vi "loadM100CRH3605MDB.vi"() -> ()   [LabVIEW 2012]
uses:
  <vilib>/addons/database/Connection.llb/DB Tools Open Connec (Path).vi
  <vilib>/addons/database/Connection.llb/Conn Execute.vi
  <vilib>/addons/database/Recordset.llb/Rec Destroy - Connection.vi
  <vilib>/addons/database/Connection.llb/DB Tools Open Connec (String).vi
  <vilib>/addons/database/Recordset.llb/Rec Fetch Recordset Data (R).vi
  <vilib>/addons/database/_DB Variant To Data/Database Variant To Data.xnode
  <vilib>/addons/database/NI_Database_API.lvlib
panel:
  out "String":string
  out "concatenated string":string
  out "error out 2":errorcluster
  out "text":string
  in  "path":path=path "C:/temp/mdb"
  out "filenames":string[](array[string])
  out "error out":errorcluster
  in  "Cluster":T1
  out "recordset data":variant[][](array[variant])
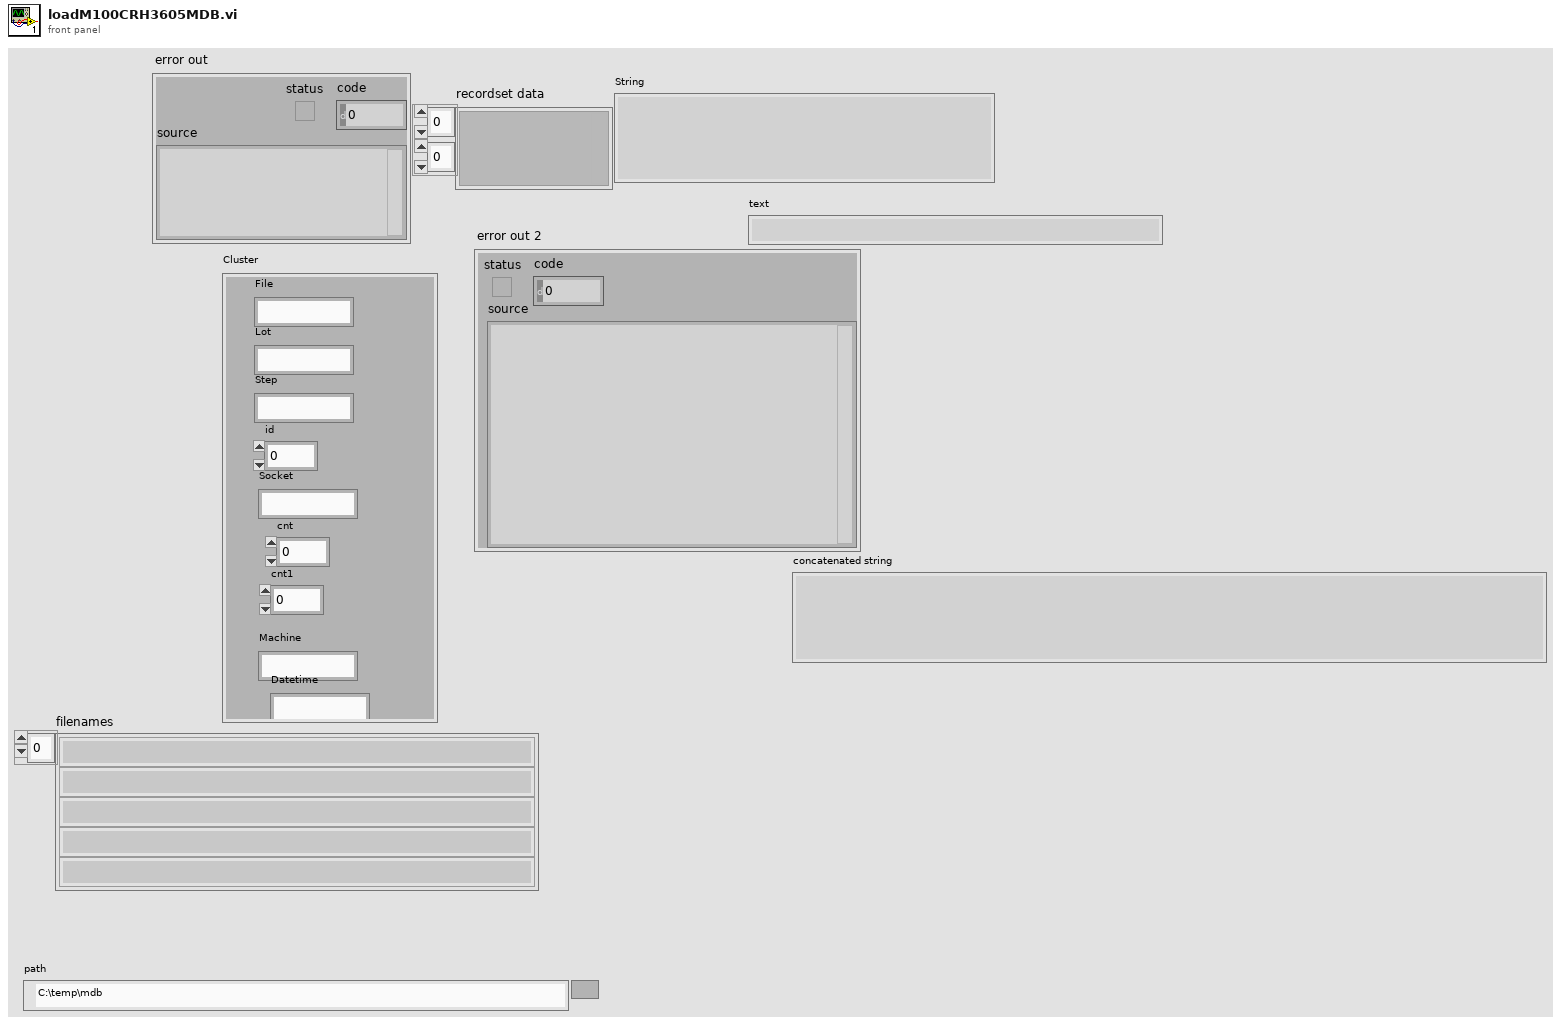
[diagram p1: front panel]
types:
  T1 = cluster{"File":string, "Lot ":string, "Step ":string, "id":dbl, "Socket":string, "cnt":dbl, "cnt1":dbl, "Machine":string, "Datetime":string}
  T2 = typedef "NI_Database_API.lvlib/Conn ObjectReference.ctl" = refnum<k1>
  T3 = typedef "NI_Database_API.lvlib/Rec ObjectReference.ctl" = refnum<k1>
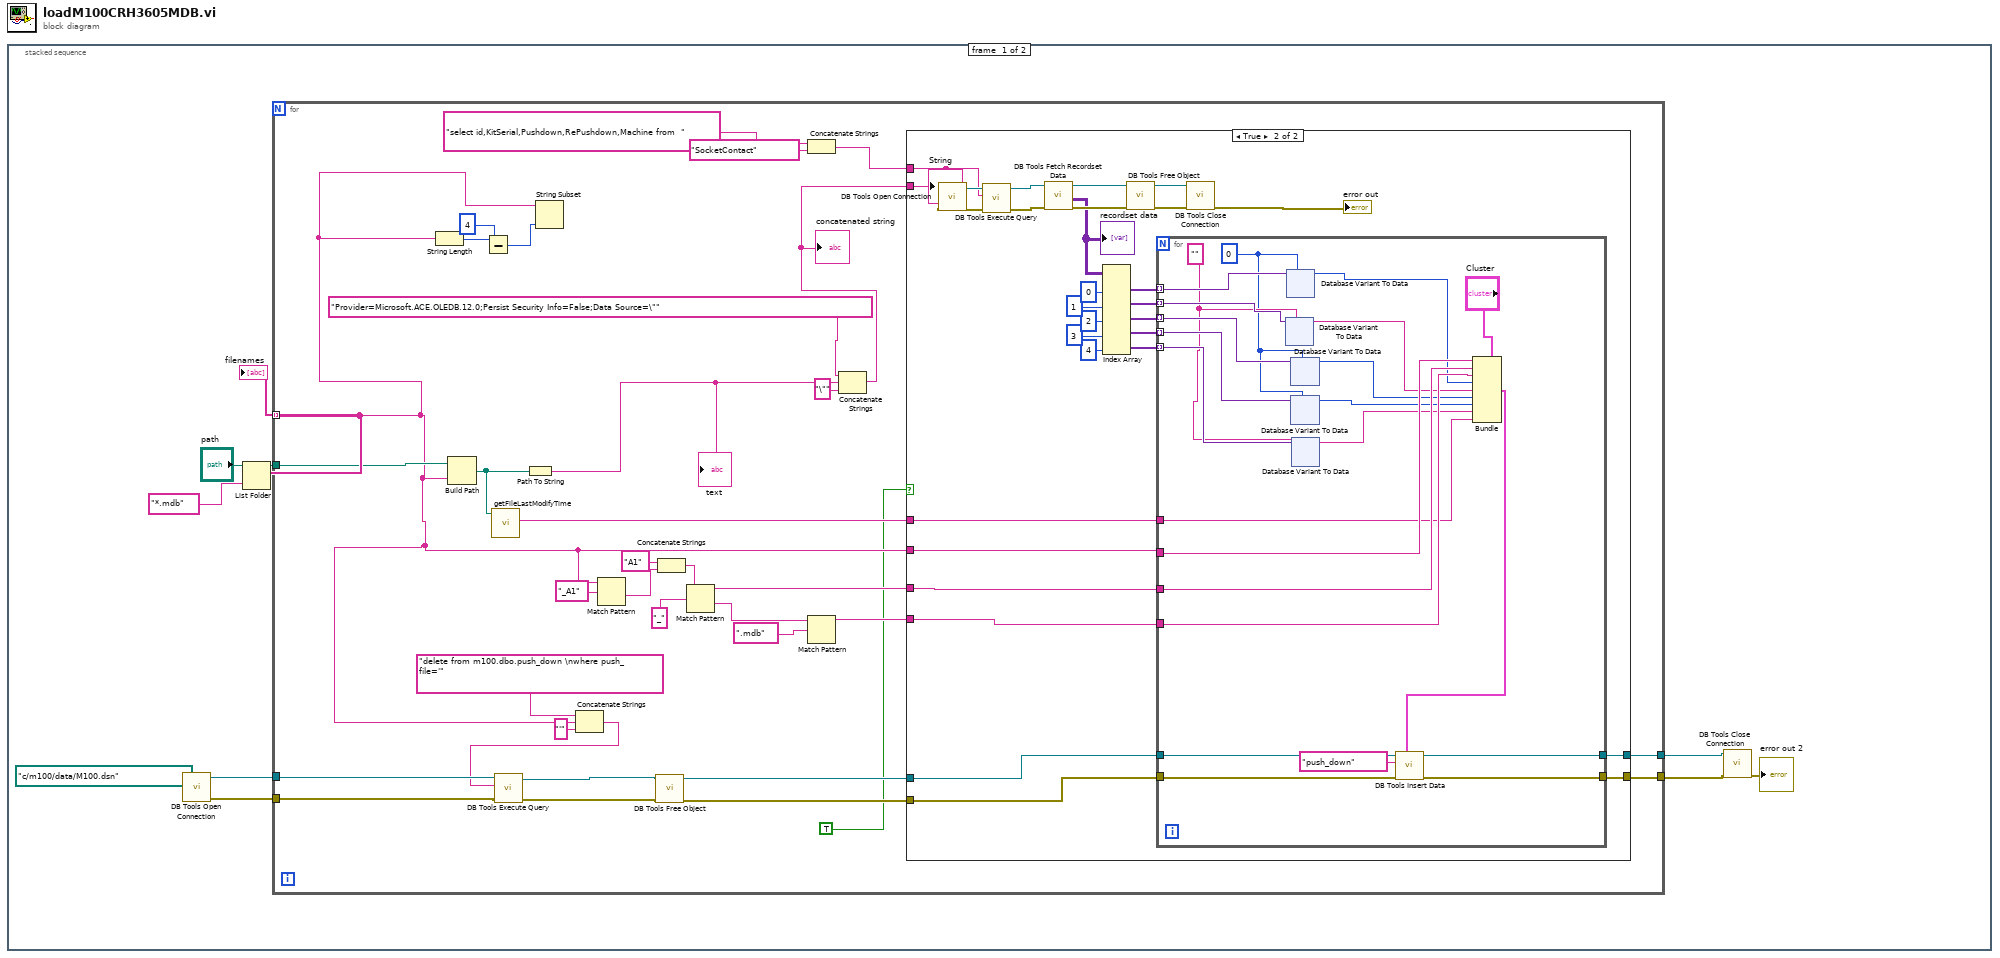
[diagram p0: block diagram]
diagram:
  n1 = stacked-sequence {
    frame #0 {
      n2 = call-poly <vilib>:"DB Tools Open Connection.vi"("connection information"=path "c:/m100/data/M100.dsn") -> ("error out"=w4:errorcluster, "connection reference"=w5:T2)  [unwired: 7 in]
      n3 = List Folder(path="path", pattern="*.mdb") -> (path out=w7:path, filenames=w8:string[])  [unwired: 2 in, 2 out]
      "filenames" <- w8
      n4 = for {
        tunnel: w8 -> [w28] mode=indexing
        tunnel: w7 -> [w43]
        tunnel: w5 -> [w30]
        tunnel: w4 -> [w31]
        tunnel: [w23] -> w3
        tunnel: [w22] -> w2
        n5 = String Length(string=w28) -> (length=w39:i32)
        n6 = Build Path(base path=w43, name or relative path=w28) -> (appended path=w15:path)
        n7 = Subtract(x=w39, y=4) -> (x-y=w37:i32)
        n8 = call "getFileLastModifyTime.vi"("path"=w15) -> ("date/time string"=w14:string)  [unwired: 10 in]
        n9 = Path To String(path=w15) -> (string=w42:string)
        "text" <- w42
        n10 = String Subset(string=w28, length (rest)=w37) -> ()  [unwired: 1 in, 1 out]
        n11 = Concatenate Strings("delete from m100.dbo.push_down \nwhere push_file='" ("string"), w28, "'" ("string")) -> (w26:string)
        n12 = call-poly <vilib>:"DB Tools Execute Query.vi"("error in (no error)"=w31, "SQL query"=w26, "connection reference"=w30) -> ("error out"=w11:errorcluster, "recordset reference"=w12:T3)  [unwired: 5 in]
        n13 = Match Pattern(string=w28, regular expression="_A1") -> (after substring=w18:string)  [unwired: 1 in, 3 out]
        n14 = call-poly <vilib>:"DB Tools Free Object.vi"("error in (no error)"=w11, "recordset reference"=w12) -> ("error out"=w24:errorcluster, "connection reference"=w25:T2)  [unwired: 8 in]
        n15 = Concatenate Strings("A1" ("string"), w18) -> (w17:string)
        n16 = Match Pattern(string=w17, regular expression="_") -> (before substring=w36:string, after substring=w35:string)  [unwired: 1 in, 2 out]
        n17 = Concatenate Strings("select id,KitSerial,Pushdown,RePushdown,Machine from  ", "SocketContact" ("string")) -> (w41:string)
        n18 = Match Pattern(string=w35, regular expression=".mdb") -> (before substring=w33:string)  [unwired: 1 in, 3 out]
        n19 = Concatenate Strings("Provider=Microsoft.ACE.OLEDB.12.0;Persist Security Info=False;Data Source=\"", w42, "\"" ("string")) -> (w45:string)
        "concatenated string" <- w45
        n20 = case shown="True" TRUE {
          tunnel: w45 -> [_ w58]
          tunnel: w41 -> [_ w57]
          tunnel: w36 -> [_ w56]
          tunnel: w33 -> [_ w55]
          tunnel: w28 -> [_ w54]
          tunnel: w25 -> [w47 w53]
          tunnel: w24 -> [w46 w52]
          tunnel: [w47 w51] -> w23
          tunnel: [w46 w50] -> w22
          tunnel: w14 -> [_ w48]
          frame False {
          }
          frame True {
            n21 = call-poly <vilib>:"DB Tools Open Connection.vi"("connection information"=w58) -> ("error out"=w73:errorcluster, "connection reference"=w77:T2)  [unwired: 7 in]
            n22 = call-poly <vilib>:"DB Tools Execute Query.vi"("error in (no error)"=w73, "SQL query"=w57, "connection reference"=w77) -> ("error out"=w49:errorcluster, "recordset reference"=w76:T3)  [unwired: 5 in]
            n23 = call-poly <vilib>:"DB Tools Fetch Recordset Data.vi"("error in (no error)"=w49, "recordset reference"=w76) -> ("error out"=w72:errorcluster, "recordset data"=w69:variant[][], "recordset reference out"=w75:T3)  [unwired: 3 in]
            "recordset data" <- w69
            n24 = Index Array(array=w69, index (col) #1=0 ("disabled index (col)"), index (col) #2=1 ("index (col)"), index (col) #3=2 ("index (col)"), index (col) #4=3 ("index (col)"), index (col) #5=4 ("index (col)")) -> (element #1=w63:variant[], element #2=w62:variant[], element #3=w61:variant[], element #4=w60:variant[], element #5=w59:variant[])  [unwired: 5 in]
            n25 = call-poly <vilib>:"DB Tools Free Object.vi"("error in (no error)"=w72, "recordset reference"=w75) -> ("error out"=w71:errorcluster, "connection reference"=w74:T2)  [unwired: 8 in]
            n26 = for {
              tunnel: w63 -> [w100] mode=indexing
              tunnel: w62 -> [w99] mode=indexing
              tunnel: w61 -> [w98] mode=indexing
              tunnel: w60 -> [w97] mode=indexing
              tunnel: w59 -> [w96] mode=indexing
              tunnel: w54 -> [w93]
              tunnel: w56 -> [w92]
              tunnel: w55 -> [w91]
              tunnel: w53 -> [w84]
              tunnel: w52 -> [w83]
              tunnel: [w81] -> w51
              tunnel: [w80] -> w50
              tunnel: w48 -> [w78]
              w88 = 0
              w95 = ""
              n27 = xnode "Database Variant To Data"("database variant"=w99, "type"=w95) -> ("data"=w89:string)  [unwired: 1 in, 1 out]
              n28 = xnode "Database Variant To Data"("database variant"=w100, "type"=w88) -> ("data"=w90:i32)  [unwired: 1 in, 1 out]
              n29 = xnode "Database Variant To Data"("database variant"=w98, "type"=w88) -> ("data"=w87:i32)  [unwired: 1 in, 1 out]
              n30 = xnode "Database Variant To Data"("database variant"=w97, "type"=w88) -> ("data"=w86:i32)  [unwired: 1 in, 1 out]
              n31 = xnode "Database Variant To Data"("database variant"=w96, "type"=w95) -> ("data"=w85:string)  [unwired: 1 in, 1 out]
              n32 = Bundle(cluster="Cluster", "File"=w93, "Lot"=w92, "Step"=w91, "id"=w90, "Socket"=w89, "cnt"=w87, "cnt1"=w86, "Machine"=w85, "Datetime"=w78) -> (w82:T1)
              n33 = call <vilib>:"DB Tools Insert Data.vi"("data"=w82, "error in (no error)"=w83, "table"="push_down", "connection reference"=w84) -> ("error out"=w80:errorcluster, "connection reference out"=w81:T2)  [unwired: 6 in]
            }
            n34 = call <vilib>:"DB Tools Close Connection.vi"("error in (no error)"=w71, "connection reference"=w74) -> ("error out"=→"error out":errorcluster)  [unwired: 5 in]
            "String" <- w57
          }
        }
      }
      n35 = call <vilib>:"DB Tools Close Connection.vi"("error in (no error)"=w2, "connection reference"=w3) -> ("error out"=→"error out 2":errorcluster)  [unwired: 5 in]
    }
    frame #1 {
    }
  }
